vi "cp11.vi"(3 "Sensor 4 (A/AI3 (Pin 9))":dbl, 4 "Sensor 3 (A/AI2 (Pin 7))":dbl, 5 "Sensor 2 (A/AI1 (Pin 5))":dbl, 6 "Sensor 1 (A/AI0 (Pin 3))":dbl) -> (0 "sum":dbl, 1 "y":dbl, 2 "x":dbl)   [LabVIEW 2019]
panel:
  out "L 4":dbl
  out "R 3":dbl
  out "F 2":dbl
  out "B":dbl
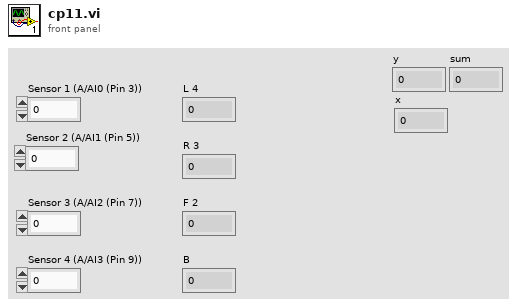
[diagram p1: front panel]
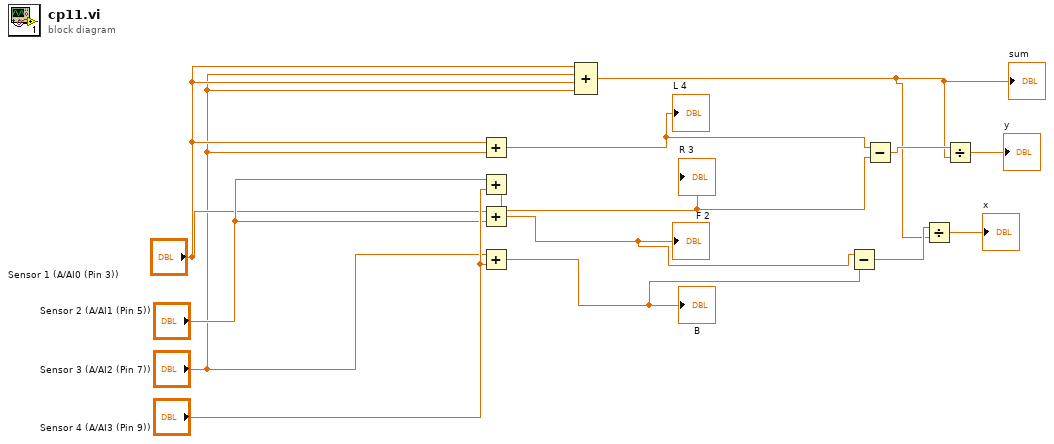
[diagram p0: block diagram]
diagram:
  n1 = Add(x="Sensor 1 (A/AI0 (Pin 3))", y="Sensor 3 (A/AI2 (Pin 7))") -> (x+y=w9:dbl)
  "L 4" <- w9
  n2 = Add(x="Sensor 2 (A/AI1 (Pin 5))", y="Sensor 4 (A/AI3 (Pin 9))") -> (x+y=w8:dbl)
  "R 3" <- w8
  n3 = Add(x="Sensor 1 (A/AI0 (Pin 3))", y="Sensor 2 (A/AI1 (Pin 5))") -> (x+y=w6:dbl)
  "F 2" <- w6
  n4 = Add(x="Sensor 3 (A/AI2 (Pin 7))", y="Sensor 4 (A/AI3 (Pin 9))") -> (x+y=w5:dbl)
  "B" <- w5
  n5 = Compound Arithmetic op=ADD("Sensor 1 (A/AI0 (Pin 3))", "Sensor 3 (A/AI2 (Pin 7))", "Sensor 1 (A/AI0 (Pin 3))", "Sensor 3 (A/AI2 (Pin 7))") -> (w3:dbl)
  "sum" <- w3
  n6 = Subtract(x=w6, y=w5) -> (x-y=w4:dbl)
  n7 = Subtract(x=w9, y=w8) -> (x-y=w7:dbl)
  n8 = Divide(x=w4, y=w3) -> (x/y=→"x":dbl)
  n9 = Divide(x=w7, y=w3) -> (x/y=→"y":dbl)
